vi "executeCommands.vi"(11 "States Enum":T1) -> ()   [LabVIEW 2017]
uses:
  Implementation/Intake Operations.ctl
panel:
  # "input state enum"
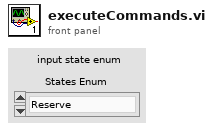
[diagram p1: front panel]
types:
  T1 = typedef "Intake Operations.ctl" = enum16{"Reserve", "setSetpoint", "feed", "spit"}
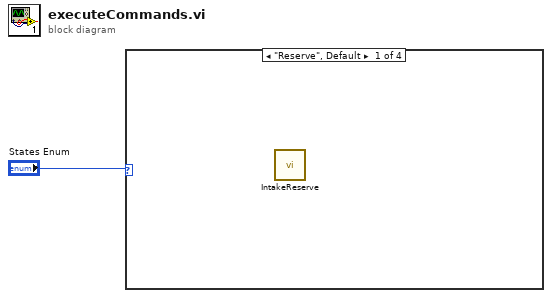
[diagram p0: block diagram]
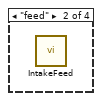
[diagram p2: hidden frame]
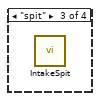
[diagram p3: hidden frame]
diagram:
  n1 = case shown="\"Reserve\", Default" "States Enum" {
    frame "Reserve", Default {
      n2 = call "IntakeReserve.vi"() -> ()  [unwired: 11 in, 1 out]
    }
    frame "feed" {
      n3 = call "IntakeFeed.vi"() -> ()  [unwired: 11 in, 1 out]
    }
    frame "spit" {
      n4 = call "IntakeSpit.vi"() -> ()  [unwired: 11 in, 1 out]
    }
    frame "setSetpoint" {
    }
  }
